vi "User Facing Message Manager.vi"(8 "error in":errorcluster, 9 "Variable Msg":string[](array[string]), 11 "User Facing Msg":T1) -> (0 "error out":errorcluster, 1 "Sub User Facing Msg Out":string, 3 "User Facing Msg Out":string)   [LabVIEW 2020, in "GUCalibration2.lvlib"]
uses:
  GUCalibration2.lvlib
  Controls/User Facing Msg Enum.ctl
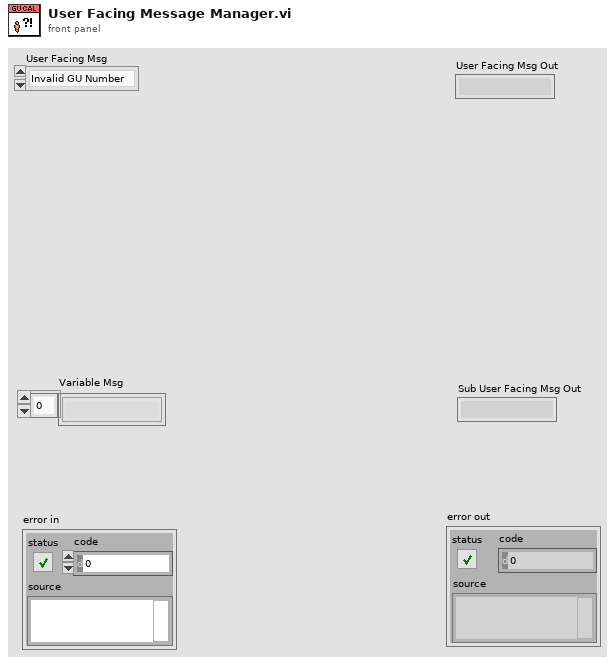
[diagram p1: front panel]
types:
  T1 = typedef "GUCalibration2.lvlib/User Facing Msg Enum.ctl" = enum16{"Invalid GU Number", "Select More GU", "Exceptional Lot End", "Not All Sites Test", "GU Arrange Error", "Put GU In Sites", "No Cal Site Offset Msg"}
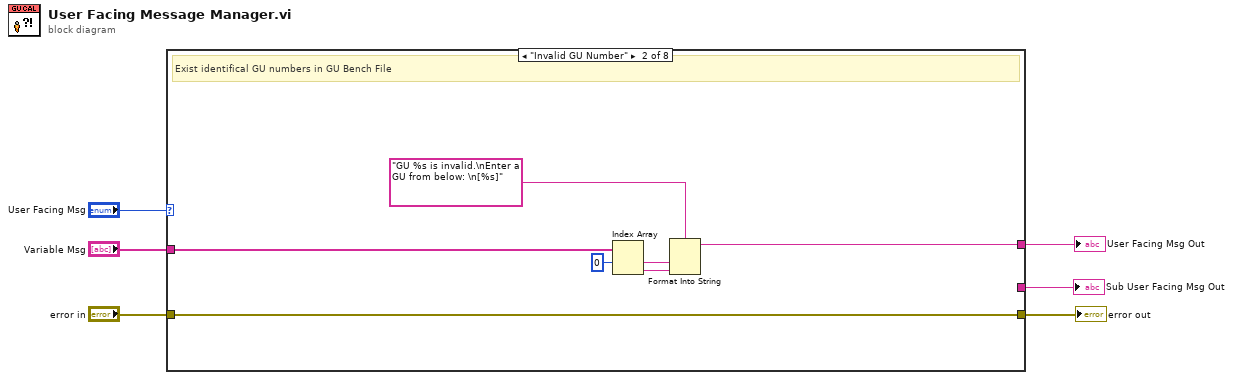
[diagram p0: block diagram]
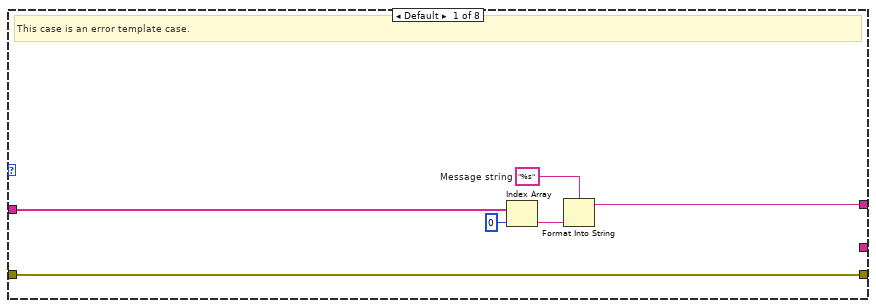
[diagram p2: hidden frame]
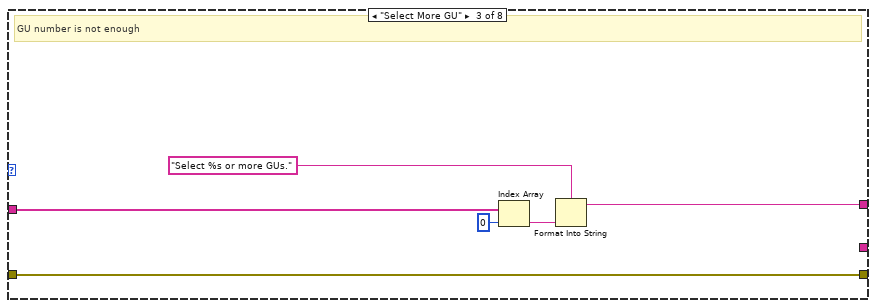
[diagram p3: hidden frame]
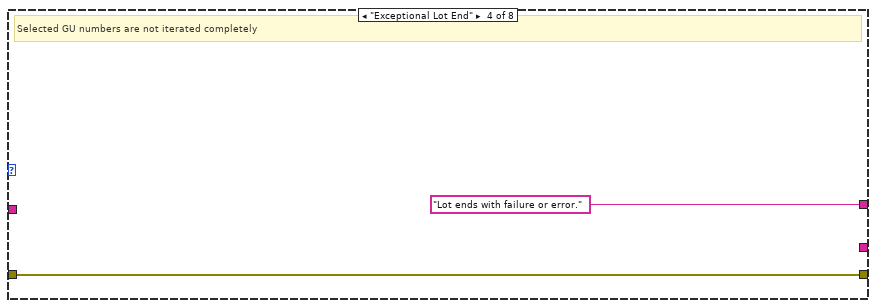
[diagram p4: hidden frame]
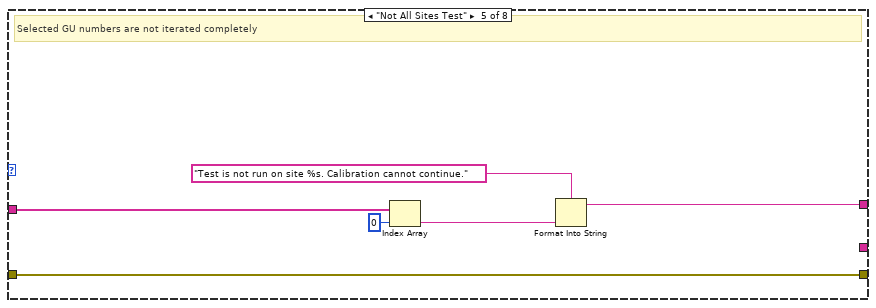
[diagram p5: hidden frame]
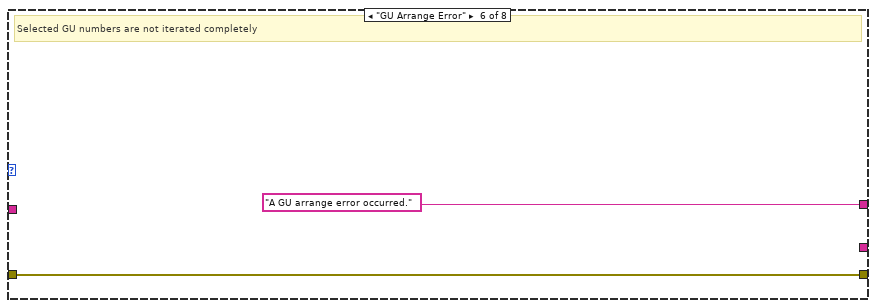
[diagram p6: hidden frame]
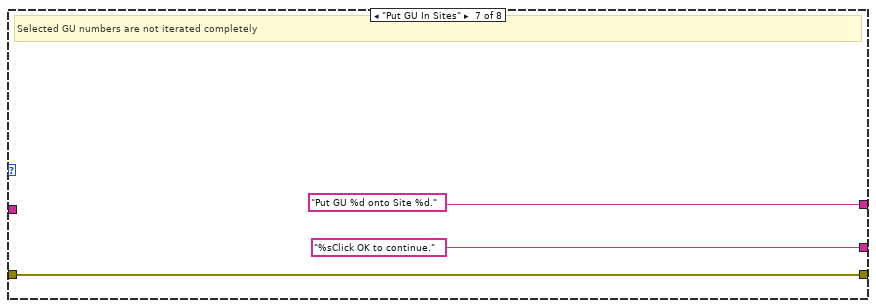
[diagram p7: hidden frame]
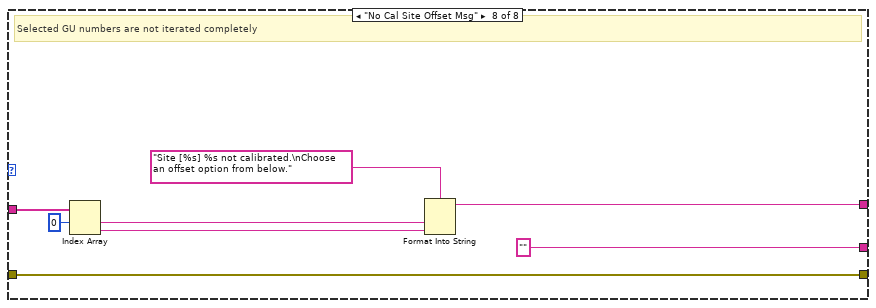
[diagram p8: hidden frame]
diagram:
  n1 = case shown="\"Invalid GU Number\"" "User Facing Msg" {
    tunnel: [w8 w16 w25 w27 w33 w35 w38 w46] -> w6
    tunnel: "error in" -> [w8 w16 w25 w27 w33 w35 w38 w46]
    tunnel: "Variable Msg" -> [w11 w19 w22 _ w31 _ _ w44]
    tunnel: [w7 w13 w20 "Lot ends with failure or error." w28 "A GU arrange error occurred." "Put GU %d onto Site %d." w39] -> w2
    tunnel: [_ _ _ _ _ _ "%sClick OK to continue." ""] -> w1
    frame Default {
      w12 = "%s"  # Message string
      # "This case is an error template case."
      n2 = Index Array(array=w11, index=0) -> (element=w9:string)
      n3 = Format Into String(format string=w12, w9) -> (resulting string=w7:string)  [unwired: 2 in, 1 out]
    }
    frame "Invalid GU Number" {
      # "Exist identifical GU numbers in GU Bench File"
      n4 = Index Array(array=w19, index #1=0 ("index")) -> (element #1=w17:string, element #2=w14:string)  [unwired: 1 in]
      n5 = Format Into String(format string="GU %s is invalid.\nEnter a GU from below: \n[%s]", w17, w14) -> (resulting string=w13:string)  [unwired: 2 in, 1 out]
    }
    frame "Select More GU" {
      # "GU number is not enough"
      n6 = Index Array(array=w22, index=0) -> (element=w21:string)
      n7 = Format Into String(format string="Select %s or more GUs.", w21) -> (resulting string=w20:string)  [unwired: 2 in, 1 out]
    }
    frame "Exceptional Lot End" {
      # "Selected GU numbers are not iterated completely"
    }
    frame "Not All Sites Test" {
      # "Selected GU numbers are not iterated completely"
      n8 = Index Array(array=w31, index=0) -> (element=w29:string)
      n9 = Format Into String(format string="Test is not run on site %s. Calibration cannot continue.", w29) -> (resulting string=w28:string)  [unwired: 2 in, 1 out]
    }
    frame "GU Arrange Error" {
      # "Selected GU numbers are not iterated completely"
    }
    frame "Put GU In Sites" {
      # "Selected GU numbers are not iterated completely"
    }
    frame "No Cal Site Offset Msg" {
      # "Selected GU numbers are not iterated completely"
      n10 = Index Array(array=w44, index #1=0 ("index")) -> (element #1=w41:string, element #2=w40:string)  [unwired: 1 in]
      n11 = Format Into String(format string="Site [%s] %s not calibrated.\nChoose an offset option from below.", w41, w40) -> (resulting string=w39:string)  [unwired: 2 in, 1 out]
    }
  }
  "error out" <- w6
  "User Facing Msg Out" <- w2
  "Sub User Facing Msg Out" <- w1
